vi "build.flowToVarient.vi"(11 "Flow Element":T1) -> (0 "error out":errorcluster, 3 "instructions out":variant[](array[variant])=[variant("stepDoutString"=variant(string ""), "stepFunction"=variant(enum16{"__NO-OP", "_DELAY_LOAD", "_DELAY_COMPARE", "_COMPARE", "_JUMP", "_FINISH", "CLK_COMPARE", "PROC_START", "PROC_STOP", "PROC_ISRUN_IF_OFF", "PROC_ISRUN_LOAD", "_IO_READ_IN", "_IO_WRITE_DOUT", "_IO_COMPARE", "Q_OPEN", "Q_WRITE", "Q_READ"} enum."_IO_WRITE_DOUT"), "stepIoPointer"=variant(string ""), "stepLabel"=variant(string ""), "stepPath"=variant(string ""))])   [LabVIEW 2024]
uses:
  controls/UiStepBuilder.ctl
  controls/type.step-builder.ctl
  controls/typeStepVarients.ctl
  controls/type.StepFunction.ctl
  Polymorphics/variantCtrlStepFunction.vi
  Polymorphics/variantCtrlSetpoint.vi
  Polymorphics/variantCtrlString.vi
  Polymorphics/variantCtrlNumber.vi
  proc.util.validateParamExist.vi
  <vilib>/Utility/error.llb/Clear Errors.vi
  <vilib>/Utility/error.llb/Trim Whitespace.vi
  <vilib>/Utility/error.llb/Trim Whitespace One-Sided.vi
  util.error.create.vi
  Polymorphics/variantCtrlStepPointer.vi
  Polymorphics/variantCtrlStepUserMessage.vi
  Polymorphics/variantCtrlStepPath.vi
  <vilib>/Utility/miscctls.llb/LVPointTypeDef.ctl
panel:
  out "format string":string
  # "UNIT-CHECK(UNIT_INDEX)"
  # "UNIT-DOSE(UNIT_INDEX,DOSE_PUNP,DOSE_TIME)"
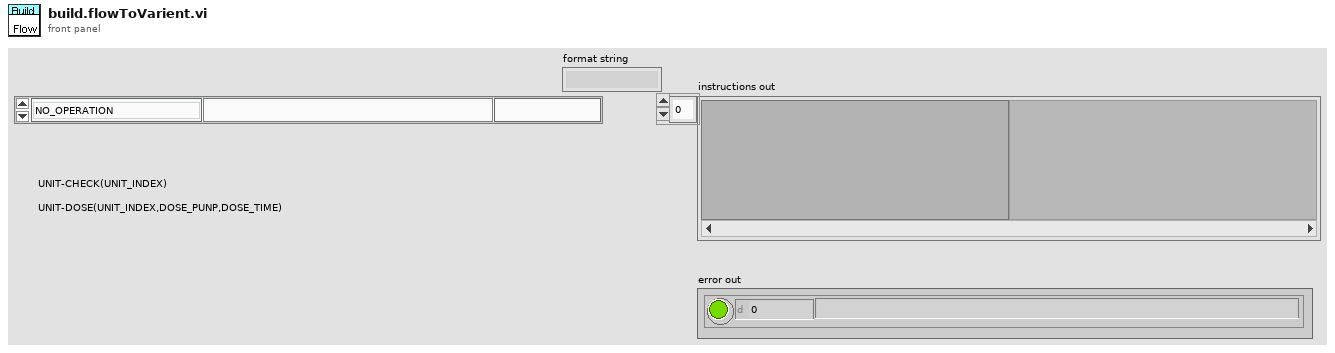
[diagram p1: front panel]
types:
  T1 = typedef "UiStepBuilder.ctl" = cluster{"Step Function":T2, "ParamString":string, "Step Label":string}
  T2 = typedef "type.step-builder.ctl" = enum16{"NO_OPERATION", "DELAY-JUMP", "DELAY", "JUMP", "COMPLETE", "SCHEDULER", "IRR-CHECK", "UNIT-CHECK", "UNIT-SAMPLE", "UNIT-DOSE", "LOG-REPORT", "LOG-MESSAGE", "IO-READ", "IO-READ-MANY", "IO-WRITE", "IO-COMPARE-OUT", "IO-COMPARE-IN", "PROC-START", "PROC-STOP", "PROC-LOAD", "PROC-IS-COMPLETED", "RECORD-MOVE", "GET-RH", "GET-UV", "GET-WD", "GET-WS", "OCS-CHECK", "OCS-RECORD"}
  T3 = typedef "typeStepVarients.ctl" = enum16{"stepNameID", "stepFunction", "stepReport", "stepSetpoint", "stepPointer", "stepProcPointer", "stepIoPointer", "stepIoValue", "stepFilePointer", "stepMessage", "stepTimeString", "stepNumReg", "stepStrReg", "stepSeconds", "stepUnitDoseParams", "stepUnitIndex"}
  T4 = typedef "LVPointTypeDef.ctl" = cluster{"Horizontal":i16, "Vertical":i16}
  T5 = typedef "type.StepFunction.ctl" = enum16{"__NO-OP", "_DELAY_LOAD", "_DELAY_COMPARE", "_JUMP", "_COMPLETE", "_COMPARE", "_LOG_MESSAGE", "_LOG_LAST_REPORT", "_SCHEDULE", "_SCHED_DAILY", "CLK_COMPARE", "PROC_START", "PROC_STOP", "PROC_LOAD", "PROC_COMPLETION_CHECK", "PROC_COMPLETION_LOAD", "_IO_READ", "_IO_READ_MANY", "_IO_WRITE", "_IO_WRITE_BY_REG", "_IO_GET_OUTPUT", "_OCS_CHECK", "_OCS_RECORD", "_GET_RH", "_GET_ACC_UV", "_GET_WD", "_GET_WS", "_REC_DELETE", "_REC_MOVE", "_REC_COPY", "_IRR_CHECK", "UNIT_CHECK", "UNIT_SAMPLE", "UNIT_DOSE"}
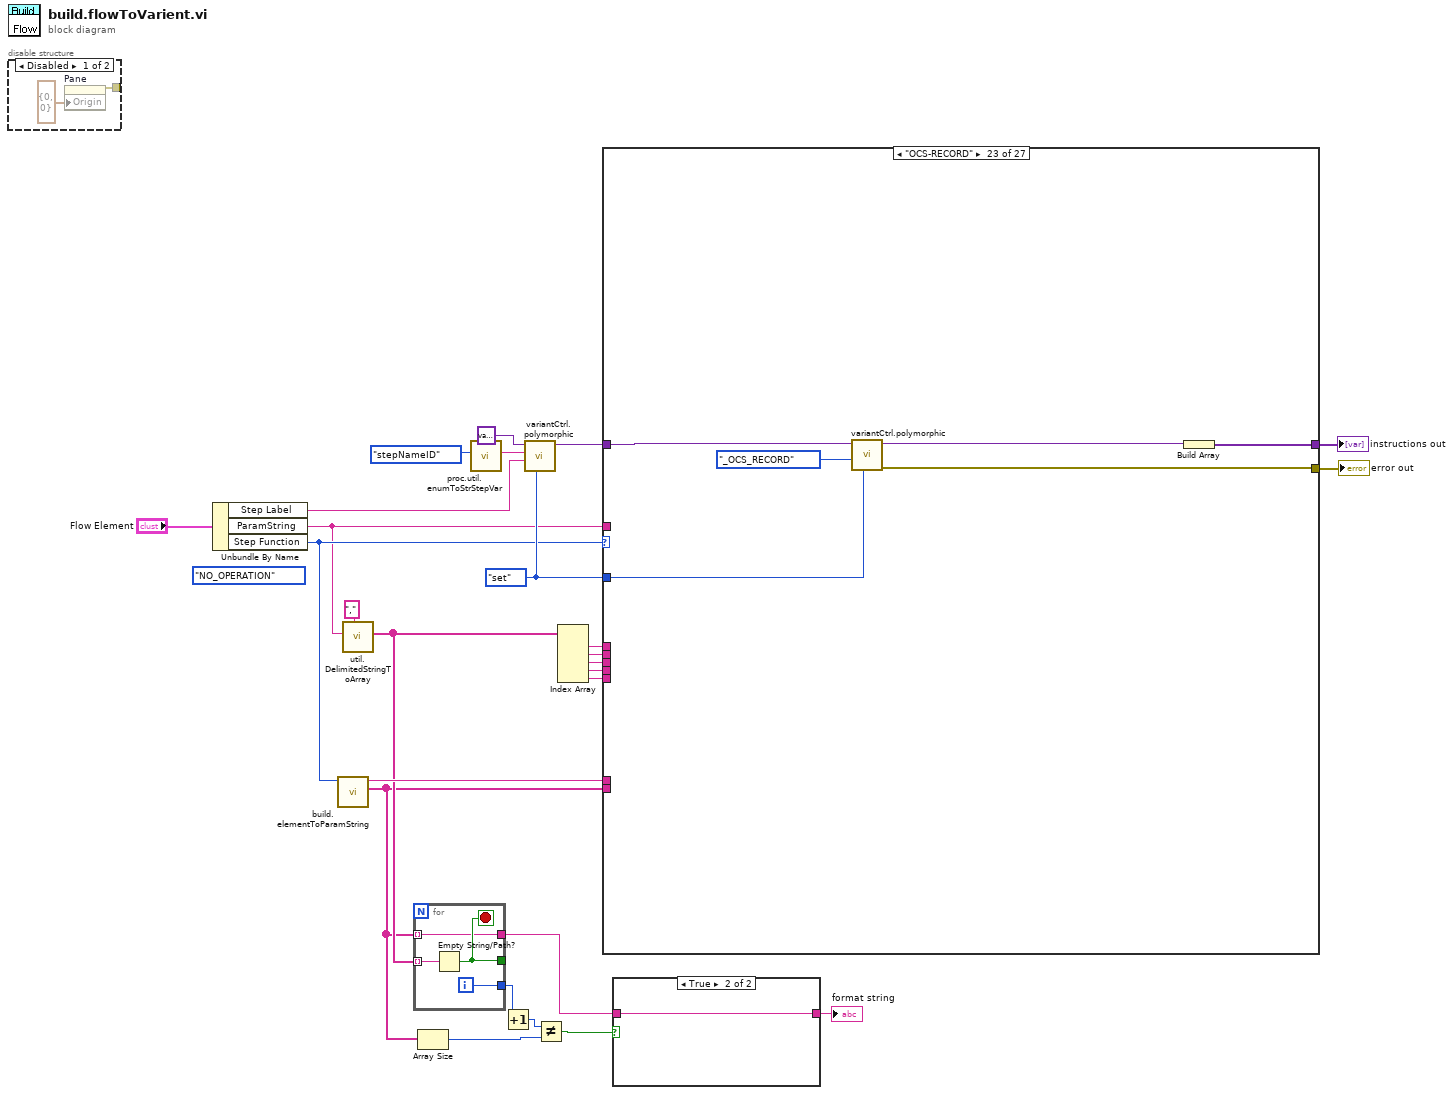
[diagram p0: block diagram]
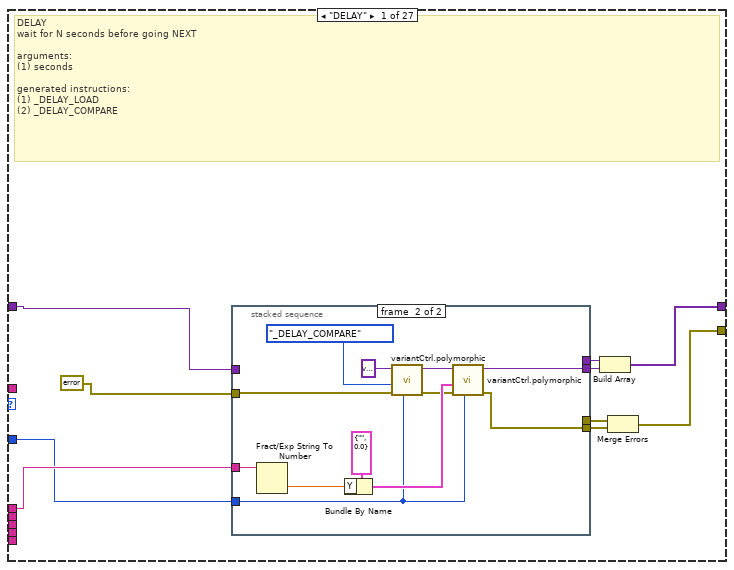
[diagram p3: hidden frame]
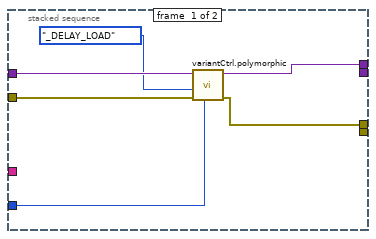
[diagram p4: hidden frame]
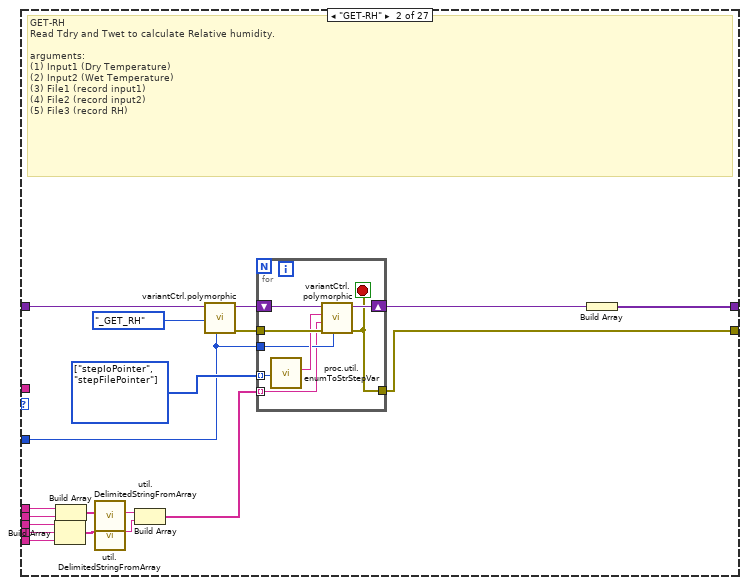
[diagram p5: hidden frame]
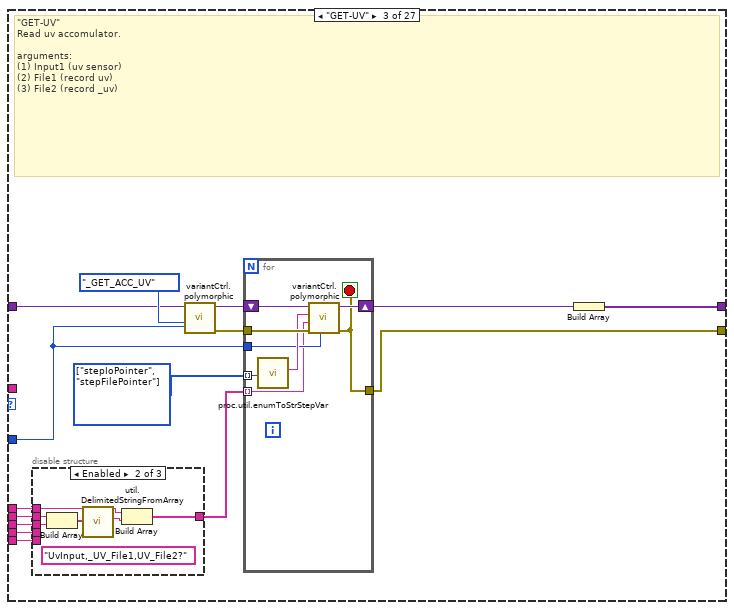
[diagram p6: hidden frame]
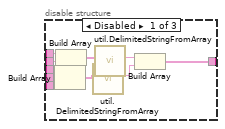
[diagram p7: hidden frame]
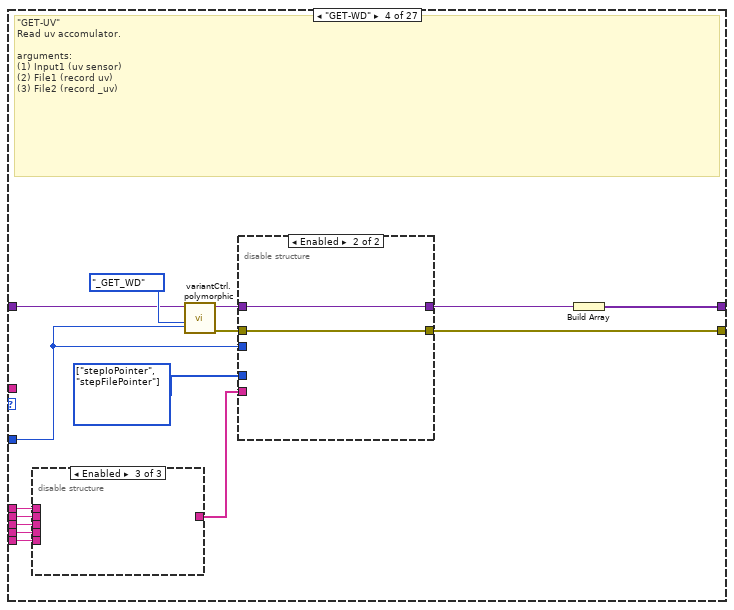
[diagram p9: hidden frame]
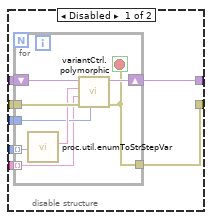
[diagram p10: hidden frame]
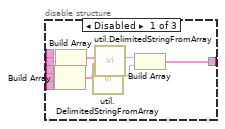
[diagram p11: hidden frame]
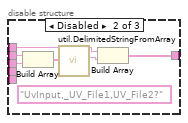
[diagram p12: hidden frame]
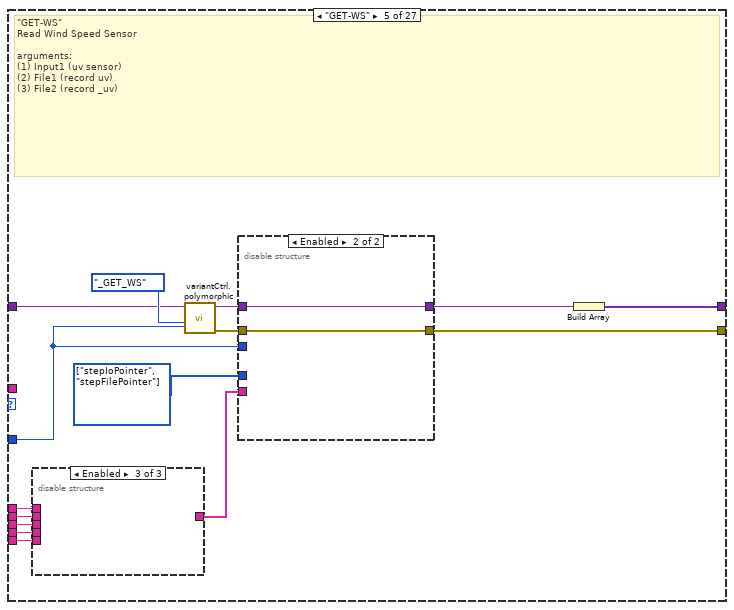
[diagram p13: hidden frame]
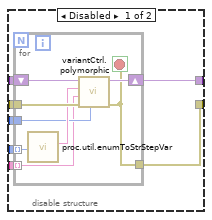
[diagram p14: hidden frame]
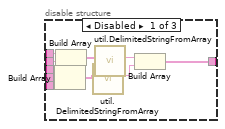
[diagram p15: hidden frame]
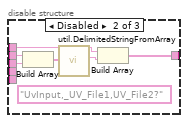
[diagram p16: hidden frame]
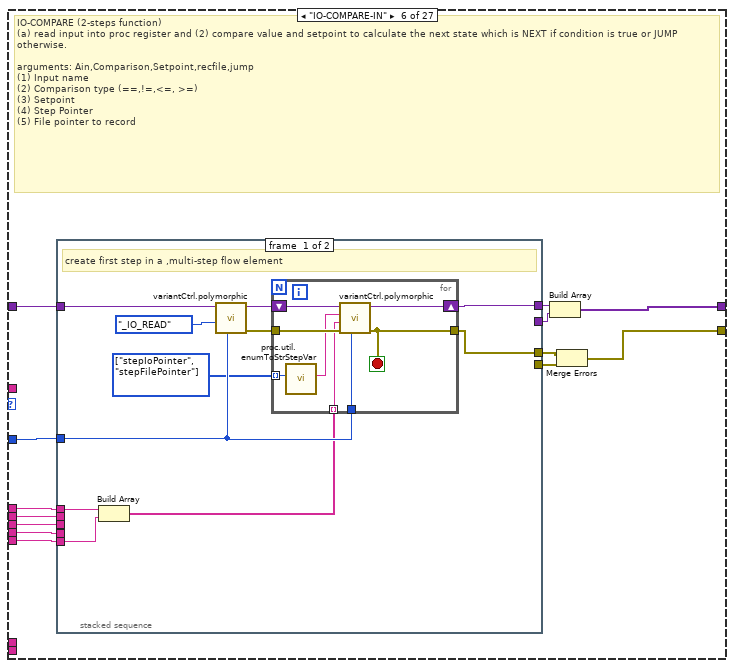
[diagram p17: hidden frame]
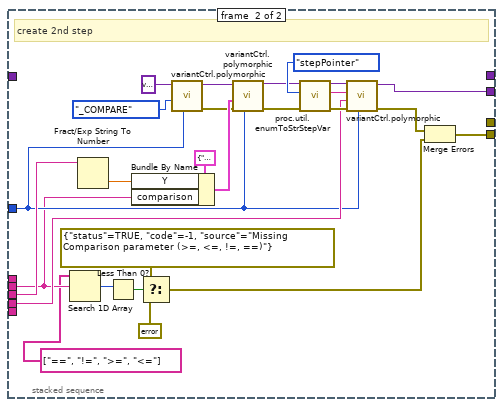
[diagram p18: hidden frame]
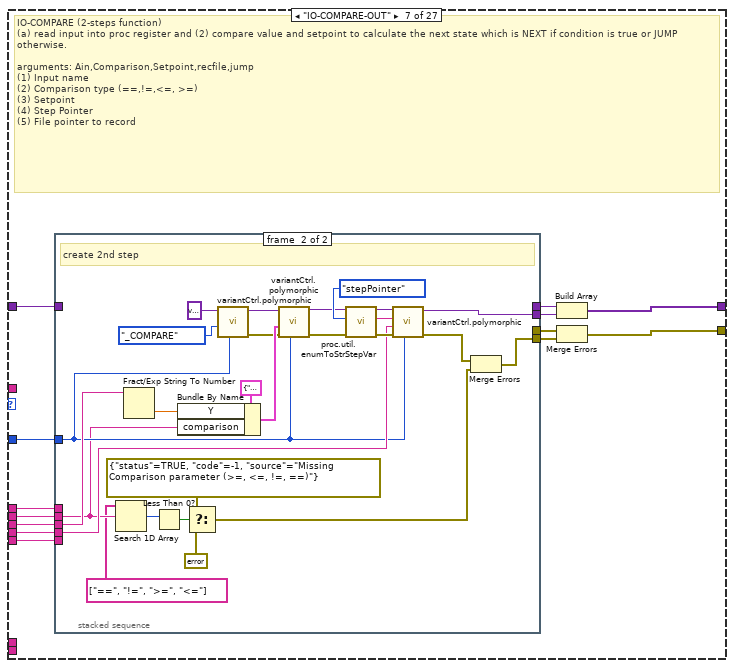
[diagram p19: hidden frame]
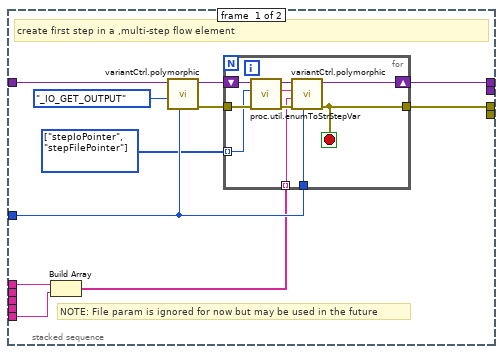
[diagram p20: hidden frame]
diagram:
  (unwired) type.step-builder."NO_OPERATION" ("Step Function")
  w16 = enum16{"get", "set"}."set" ("get/set")
  n1 = disable-structure shown="Disabled" {
    disable-tunnel: [w27 _] -> _
    frame Disabled {
      n2 = property on="Pane" class="Pane"("Origin"=T4 {"Horizontal"=0, "Vertical"=0}) -> (error out=w27:errorcluster)  [unwired: 2 in, 1 out]
    }
    frame Enabled {
    }
  }
  n3 = Unbundle By Name("Flow Element") -> ("Step Label"=w23:string, "ParamString"=w1:string, "Step Function"=w12:T2)
  n4 = call "build.elementToParamString.vi"("UiStepFunction"=w12) -> ("params"=w6:string[], "source"=w11:string)  [unwired: 9 in]
  n5 = call "util.DelimitedStringToArray.vi"("delimiter (,)"=",", "delimitaed string"=w1) -> ("array out"=w10:string[])  [unwired: 9 in]
  n6 = for {
    tunnel: w10 -> [w32] mode=indexing
    tunnel: [w31] -> w9
    tunnel: [w30] -> _
    tunnel: w6 -> [w29] mode=indexing
    tunnel: [w29] -> w4
    i -> [w31]
    stop <- w30 stop-if-true
    n7 = Empty String/Path?(string/path=w32) -> (empty?=w30:bool)
  }
  n8 = Array Size(array=w6) -> (size(s)=w8:i32)
  n9 = call "proc.util.enumToStrStepVar.vi"("Step var"=typeStepVarients."stepNameID") -> ("String"=w20:string)  [unwired: 10 in]
  n10 = Increment(x=w9) -> (x+1=w7:i32)
  n11 = call-poly "variantCtrl.polymorphic.vi"("menu in (get)"=w16, "String Value"=w23, "name in"=w20, "Step in"=variant ("stepElement _DELAY_LOAD")) -> ("Step out"=w19:variant)  [unwired: 4 in, 3 out]
  n12 = Not Equal?(x=w7, y=w8) -> (x != y?=w5:bool)
  n13 = Index Array(array=w10) -> (element #1=w18:string, element #2=w17:string, element #3=w15:string, element #4=w14:string, element #5=w13:string)  [unwired: 5 in]
  n14 = case shown="\"OCS-RECORD\"" w12 {
    selector: w12 -> [_ _ _ _ _ _ _ _ _ _ _ _ _ _ _ _ _ _ _ _ _ _ _ _ _ _ w655]
    tunnel: [w39 w79 w102 w141 w189 w235 w291 w341 w366 w398 w415 w421 w433 w450 w459 w490 w501 w512 w528 w555 w569 w585 w591 w603 w617 w647 variant[] []] -> w26
    tunnel: [w42 w75 w97 w136 w184 w234 w290 w340 w365 w397 w408 w416 w424 w446 w454 w483 w495 w505 w523 w554 w568 w582 w588 w602 w616 w649 w652] -> w25
    tunnel: w19 -> [w41 w72 w94 w133 w181 w233 w289 w337 w362 w395 w411 w419 w432 w449 w453 w480 w491 w502 w520 w553 w567 w584 w590 w601 w615 w648 _]
    tunnel: w16 -> [w33 w74 w96 w135 w183 w232 w288 w339 w364 _ w410 w418 w423 w448 w452 w482 w494 w504 w522 w552 w566 w583 w589 w600 w614 w628 _]
    tunnel: w18 -> [w40 w73 w95 w134 w182 w231 w287 w338 w363 w396 w407 _ w428 w442 w451 w481 w492 w503 w521 w545 w557 _ _ _ w605 w629 _]
    tunnel: w17 -> [_ w70 w92 w131 w179 w230 w286 w335 _ w392 _ _ w422 _ _ _ _ _ w518 _ _ _ _ _ _ w646 _]
    tunnel: w15 -> [_ w67 w91 w130 w178 w229 w285 _ _ w391 _ _ _ _ _ _ _ _ w517 _ _ _ _ _ _ w645 _]
    tunnel: w14 -> [_ w66 w90 w129 w177 w228 w284 _ _ _ _ _ _ _ _ _ _ _ w516 _ _ _ _ _ _ _ _]
    tunnel: w13 -> [_ w65 w89 w128 w176 w227 w283 _ _ _ _ _ _ _ _ _ _ _ w515 _ _ _ _ _ _ _ _]
    tunnel: w11 -> [_ _ _ _ _ _ _ _ _ _ _ _ _ _ _ _ _ _ _ _ _ _ _ _ _ _ _]
    tunnel: w6 -> [_ _ _ _ _ _ _ _ _ _ _ _ _ _ _ _ _ _ _ _ _ _ _ _ _ _ _]
    tunnel: w1 -> [_ _ _ _ _ _ _ _ _ _ _ _ _ _ _ _ _ _ _ _ _ _ _ w592 _ _ _]
    frame "DELAY" {
      # "DELAY\nwait for N seconds before going NEXT\n\narguments:\n(1) seconds\n\ngenerated instructions:\n(1) _DELAY_LOAD\n(2) _DELAY_COMPARE"
      n15 = stacked-sequence {
        tunnel: [w46 _] -> w37
        tunnel: [_ w51] -> w36
        tunnel: [_ w59] -> w35
        tunnel: [w45 _] -> w34
        tunnel: w40 -> [_ w58]
        tunnel: w41 -> [w48 _]
        tunnel: w33 -> [w47 w54]
        tunnel: errorcluster {"status"=FALSE, "code"=0, "source"=""} ("error in") -> [w43 w49]
        frame #0 {
          n16 = call-poly "variantCtrl.polymorphic.vi"("menu in (get)"=w47, "error in"=w43, "StepFunction"=type.StepFunction."_DELAY_LOAD" ("Operation out"), "variant in"=w48) -> ("error out"=w45:errorcluster, "variant out"=w46:variant)  [unwired: 4 in, 2 out]
        }
        frame #1 {
          n17 = Fract/Exp String To Number(string=w58) -> (number=w57:dbl)  [unwired: 3 in, 1 out]
          n18 = Bundle By Name(cluster=cluster{"comparison":string, "Y":dbl} {"comparison"="", "Y"=0.0} ("setpoint 2"), "Y"=w57) -> (w60:cluster{"comparison":string, "Y":dbl})
          n19 = call-poly "variantCtrl.polymorphic.vi"("menu in (get)"=w54, "error in"=w49, "StepFunction"=type.StepFunction."_DELAY_COMPARE" ("Operation out"), "variant in"=variant ("stepElement _DELAY_LOAD")) -> ("error out"=w55:errorcluster, "variant out"=w56:variant)  [unwired: 4 in, 2 out]
          n20 = call-poly "variantCtrl.polymorphic.vi"("get/set"=w54, "error in"=w55, "setpoint"=w60, "procElement in in"=w56) -> ("error out"=w59:errorcluster, "procElement out"=w51:variant)  [unwired: 4 in, 2 out]
        }
      }
      n21 = Build Array(w37, w36) -> (w39:variant[])
      n22 = Merge Errors(w34, w35) -> (w42:errorcluster)
    }
    frame "GET-RH" {
      w76 = T3[] [enum."stepIoPointer", enum."stepFilePointer"] items=["stepNameID", "stepFunction", "stepReport", "stepSetpoint", "stepPointer", "stepProcPointer", "stepIoPointer", "stepIoValue", "stepFilePointer", "stepMessage", "stepTimeString", "stepNumReg", "stepStrReg", "stepSeconds", "stepUnitDoseParams", "stepUnitIndex"] ("Step var")
      # "GET-RH\nRead Tdry and Twet to calculate Relative humidity.\n\narguments:\n(1) Input1 (Dry Temperature)\n(2) Input2 (Wet Temperature)\n(3) File1 (record input1)\n(4) File2 (record input2)\n(5) File3 (record RH)"
      n23 = Build Array(w67, w66, w65) -> (w64:string[])
      n24 = Build Array(w73, w70) -> (w69:string[])
      n25 = call "util.DelimitedStringFromArray.vi"("params array in"=w69) -> ("delimited string out"=w68:string)  [unwired: 10 in]
      n26 = call "util.DelimitedStringFromArray.vi"("params array in"=w64) -> ("delimited string out"=w62:string)  [unwired: 10 in]
      n27 = Build Array(w68, w62) -> (w63:string[])
      n28 = call-poly "variantCtrl.polymorphic.vi"("menu in (get)"=w74, "StepFunction"=type.StepFunction."_GET_RH" ("Operation out"), "variant in"=w72) -> ("error out"=w78:errorcluster, "variant out"=w77:variant)  [unwired: 5 in, 2 out]
      n29 = for {
        tunnel: w76 -> [w85] mode=indexing
        tunnel: w74 -> [w83]
        tunnel: w63 -> [w82] mode=indexing
        shift-right: [w81] -> w71
        shift-left: w77 -> [w86]
        tunnel: w78 -> [w87]
        tunnel: [w80] -> w75
        stop <- w80 stop-if-true
        n30 = call "proc.util.enumToStrStepVar.vi"("Step var"=w85) -> ("String"=w84:string)  [unwired: 10 in]
        n31 = call-poly "variantCtrl.polymorphic.vi"("menu in (get)"=w83, "error in"=w87, "String Value"=w82, "name in"=w84, "Step in"=w86) -> ("error out"=w80:errorcluster, "Step out"=w81:variant)  [unwired: 3 in, 2 out]
      }
      n32 = Build Array(w71) -> (w79:variant[])
    }
    frame "GET-UV" {
      w98 = T3[] [enum."stepIoPointer", enum."stepFilePointer"] items=["stepNameID", "stepFunction", "stepReport", "stepSetpoint", "stepPointer", "stepProcPointer", "stepIoPointer", "stepIoValue", "stepFilePointer", "stepMessage", "stepTimeString", "stepNumReg", "stepStrReg", "stepSeconds", "stepUnitDoseParams", "stepUnitIndex"] ("Step var")
      # "\"GET-UV\" \nRead uv accomulator.\n\narguments:\n(1) Input1 (uv sensor)\n(2) File1 (record uv)\n(3) File2 (record _uv)"
      n33 = disable-structure shown="Enabled" {
        disable-tunnel: w95 -> [w112 w114 _]
        disable-tunnel: w92 -> [w111 w113 _]
        disable-tunnel: w91 -> [w108 w118 _]
        disable-tunnel: w90 -> [w107 _ _]
        disable-tunnel: w89 -> [w106 _ _]
        disable-tunnel: [w104 w116 _] -> w88
        frame Disabled {
          n34 = Build Array(w108, w107, w106) -> (w105:string[])
          n35 = Build Array(w112, w111) -> (w110:string[])
          n36 = call "util.DelimitedStringFromArray.vi"("params array in"=w105) -> ("delimited string out"=w103:string)  [unwired: 10 in]
          n37 = call "util.DelimitedStringFromArray.vi"("params array in"=w110) -> ("delimited string out"=w109:string)  [unwired: 10 in]
          n38 = Build Array(w109, w103) -> (w104:string[])
        }
        frame Enabled {
          (unwired) "UvInput,_UV_File1,UV_File2?" ("source")
          n39 = Build Array(w113, w118) -> (w117:string[])
          n40 = call "util.DelimitedStringFromArray.vi"("params array in"=w117) -> ("delimited string out"=w115:string)  [unwired: 10 in]
          n41 = Build Array(w114, w115) -> (w116:string[])
        }
        frame Disabled {
        }
      }
      n42 = call-poly "variantCtrl.polymorphic.vi"("menu in (get)"=w96, "StepFunction"=type.StepFunction."_GET_ACC_UV" ("Operation out"), "variant in"=w94) -> ("error out"=w101:errorcluster, "variant out"=w100:variant)  [unwired: 5 in, 2 out]
      n43 = for {
        tunnel: w98 -> [w124] mode=indexing
        tunnel: w96 -> [w122]
        tunnel: w88 -> [w121] mode=indexing
        shift-right: [w120] -> w93
        shift-left: w100 -> [w125]
        tunnel: w101 -> [w126]
        tunnel: [w119] -> w97
        stop <- w119 stop-if-true
        n44 = call "proc.util.enumToStrStepVar.vi"("Step var"=w124) -> ("String"=w123:string)  [unwired: 10 in]
        n45 = call-poly "variantCtrl.polymorphic.vi"("menu in (get)"=w122, "error in"=w126, "String Value"=w121, "name in"=w123, "Step in"=w125) -> ("error out"=w119:errorcluster, "Step out"=w120:variant)  [unwired: 3 in, 2 out]
      }
      n46 = Build Array(w93) -> (w102:variant[])
    }
    frame "GET-WD" {
      w137 = T3[] [enum."stepIoPointer", enum."stepFilePointer"] items=["stepNameID", "stepFunction", "stepReport", "stepSetpoint", "stepPointer", "stepProcPointer", "stepIoPointer", "stepIoValue", "stepFilePointer", "stepMessage", "stepTimeString", "stepNumReg", "stepStrReg", "stepSeconds", "stepUnitDoseParams", "stepUnitIndex"] ("Step var")
      # "\"GET-UV\" \nRead uv accomulator.\n\narguments:\n(1) Input1 (uv sensor)\n(2) File1 (record uv)\n(3) File2 (record _uv)"
      n47 = disable-structure shown="Enabled" {
        disable-tunnel: w134 -> [w168 w170 _]
        disable-tunnel: w131 -> [w167 w169 _]
        disable-tunnel: w130 -> [w164 w174 _]
        disable-tunnel: w129 -> [w163 _ _]
        disable-tunnel: w128 -> [w162 _ _]
        disable-tunnel: [w160 w172 _] -> w127
        frame Disabled {
          n48 = Build Array(w164, w163, w162) -> (w161:string[])
          n49 = Build Array(w168, w167) -> (w166:string[])
          n50 = call "util.DelimitedStringFromArray.vi"("params array in"=w161) -> ("delimited string out"=w159:string)  [unwired: 10 in]
          n51 = call "util.DelimitedStringFromArray.vi"("params array in"=w166) -> ("delimited string out"=w165:string)  [unwired: 10 in]
          n52 = Build Array(w165, w159) -> (w160:string[])
        }
        frame Disabled {
          (unwired) "UvInput,_UV_File1,UV_File2?" ("source")
          n53 = Build Array(w169, w174) -> (w173:string[])
          n54 = call "util.DelimitedStringFromArray.vi"("params array in"=w173) -> ("delimited string out"=w171:string)  [unwired: 10 in]
          n55 = Build Array(w170, w171) -> (w172:string[])
        }
        frame Enabled {
        }
      }
      n56 = call-poly "variantCtrl.polymorphic.vi"("menu in (get)"=w135, "StepFunction"=type.StepFunction."_GET_WD" ("Operation out"), "variant in"=w133) -> ("error out"=w140:errorcluster, "variant out"=w139:variant)  [unwired: 5 in, 2 out]
      n57 = disable-structure shown="Enabled" {
        disable-tunnel: w140 -> [w148 w157]
        disable-tunnel: w139 -> [w147 w158]
        disable-tunnel: w137 -> [w146 _]
        disable-tunnel: [w145 w157] -> w136
        disable-tunnel: w135 -> [w144 _]
        disable-tunnel: [w143 w158] -> w132
        disable-tunnel: w127 -> [w142 _]
        frame Disabled {
          n58 = for {
            tunnel: w146 -> [w154] mode=indexing
            tunnel: w144 -> [w152]
            tunnel: w142 -> [w151] mode=indexing
            shift-right: [w150] -> w143
            shift-left: w147 -> [w155]
            tunnel: w148 -> [w156]
            tunnel: [w149] -> w145
            stop <- w149 stop-if-true
            n59 = call "proc.util.enumToStrStepVar.vi"("Step var"=w154) -> ("String"=w153:string)  [unwired: 10 in]
            n60 = call-poly "variantCtrl.polymorphic.vi"("menu in (get)"=w152, "error in"=w156, "String Value"=w151, "name in"=w153, "Step in"=w155) -> ("error out"=w149:errorcluster, "Step out"=w150:variant)  [unwired: 3 in, 2 out]
          }
        }
        frame Enabled {
        }
      }
      n61 = Build Array(w132) -> (w141:variant[])
    }
    frame "GET-WS" {
      w185 = T3[] [enum."stepIoPointer", enum."stepFilePointer"] items=["stepNameID", "stepFunction", "stepReport", "stepSetpoint", "stepPointer", "stepProcPointer", "stepIoPointer", "stepIoValue", "stepFilePointer", "stepMessage", "stepTimeString", "stepNumReg", "stepStrReg", "stepSeconds", "stepUnitDoseParams", "stepUnitIndex"] ("Step var")
      # "\"GET-WS\"  \nRead Wind Speed Sensor \n\narguments:\n(1) Input1 (uv sensor)\n(2) File1 (record uv)\n(3) File2 (record _uv)"
      n62 = disable-structure shown="Enabled" {
        disable-tunnel: w182 -> [w216 w218 _]
        disable-tunnel: w179 -> [w215 w217 _]
        disable-tunnel: w178 -> [w212 w222 _]
        disable-tunnel: w177 -> [w211 _ _]
        disable-tunnel: w176 -> [w210 _ _]
        disable-tunnel: [w208 w220 _] -> w175
        frame Disabled {
          n63 = Build Array(w212, w211, w210) -> (w209:string[])
          n64 = Build Array(w216, w215) -> (w214:string[])
          n65 = call "util.DelimitedStringFromArray.vi"("params array in"=w209) -> ("delimited string out"=w207:string)  [unwired: 10 in]
          n66 = call "util.DelimitedStringFromArray.vi"("params array in"=w214) -> ("delimited string out"=w213:string)  [unwired: 10 in]
          n67 = Build Array(w213, w207) -> (w208:string[])
        }
        frame Disabled {
          (unwired) "UvInput,_UV_File1,UV_File2?" ("source")
          n68 = Build Array(w217, w222) -> (w221:string[])
          n69 = call "util.DelimitedStringFromArray.vi"("params array in"=w221) -> ("delimited string out"=w219:string)  [unwired: 10 in]
          n70 = Build Array(w218, w219) -> (w220:string[])
        }
        frame Enabled {
        }
      }
      n71 = call-poly "variantCtrl.polymorphic.vi"("menu in (get)"=w183, "StepFunction"=type.StepFunction."_GET_WS" ("Operation out"), "variant in"=w181) -> ("error out"=w188:errorcluster, "variant out"=w187:variant)  [unwired: 5 in, 2 out]
      n72 = disable-structure shown="Enabled" {
        disable-tunnel: w188 -> [w196 w205]
        disable-tunnel: w187 -> [w195 w206]
        disable-tunnel: w185 -> [w194 _]
        disable-tunnel: [w193 w205] -> w184
        disable-tunnel: w183 -> [w192 _]
        disable-tunnel: [w191 w206] -> w180
        disable-tunnel: w175 -> [w190 _]
        frame Disabled {
          n73 = for {
            tunnel: w194 -> [w202] mode=indexing
            tunnel: w192 -> [w200]
            tunnel: w190 -> [w199] mode=indexing
            shift-right: [w198] -> w191
            shift-left: w195 -> [w203]
            tunnel: w196 -> [w204]
            tunnel: [w197] -> w193
            stop <- w197 stop-if-true
            n74 = call "proc.util.enumToStrStepVar.vi"("Step var"=w202) -> ("String"=w201:string)  [unwired: 10 in]
            n75 = call-poly "variantCtrl.polymorphic.vi"("menu in (get)"=w200, "error in"=w204, "String Value"=w199, "name in"=w201, "Step in"=w203) -> ("error out"=w197:errorcluster, "Step out"=w198:variant)  [unwired: 3 in, 2 out]
          }
        }
        frame Enabled {
        }
      }
      n76 = Build Array(w180) -> (w189:variant[])
    }
    frame "IO-COMPARE-IN" {
      # "IO-COMPARE (2-steps function)\n(a) read input into proc register and (2) compare value and setpoint to calculate the next state which is NEXT if condition is true or JUMP otherwise. \n\narguments: Ain,Comparison,Setpoint,recfile,jump\n(1) Input name\n(2) Comparison type (==,!=,<=, >=)\n(3) Setpoint\n(4) Step Pointer\n(5) File pointer to record"
      n77 = stacked-sequence {
        tunnel: [w243 _] -> w226
        tunnel: w231 -> [w244 _]
        tunnel: w233 -> [w246 _]
        tunnel: w232 -> [w245 w262]
        tunnel: w230 -> [_ w261]
        tunnel: w229 -> [_ w271]
        tunnel: w228 -> [_ w263]
        tunnel: w227 -> [w236 _]
        tunnel: [_ w257] -> w225
        tunnel: [w237 _] -> w224
        tunnel: [_ w256] -> w223
        frame #0 {
          w239 = T3[] [enum."stepIoPointer", enum."stepFilePointer"] items=["stepNameID", "stepFunction", "stepReport", "stepSetpoint", "stepPointer", "stepProcPointer", "stepIoPointer", "stepIoValue", "stepFilePointer", "stepMessage", "stepTimeString", "stepNumReg", "stepStrReg", "stepSeconds", "stepUnitDoseParams", "stepUnitIndex"] ("Step var")
          # "create first step in a ,multi-step flow element"
          n78 = Build Array(w244, w236) -> (w238:string[])
          n79 = call-poly "variantCtrl.polymorphic.vi"("menu in (get)"=w245, "StepFunction"=type.StepFunction."_IO_READ" ("Operation out"), "variant in"=w246) -> ("error out"=w242:errorcluster, "variant out"=w241:variant)  [unwired: 5 in, 2 out]
          n80 = for {
            tunnel: w239 -> [w252] mode=indexing
            tunnel: w245 -> [w250]
            tunnel: w238 -> [w249] mode=indexing
            shift-right: [w248] -> w237
            shift-left: w241 -> [w253]
            tunnel: w242 -> [w254]
            tunnel: [w247] -> w243
            stop <- w247 stop-if-true
            n81 = call "proc.util.enumToStrStepVar.vi"("Step var"=w252) -> ("String"=w251:string)  [unwired: 10 in]
            n82 = call-poly "variantCtrl.polymorphic.vi"("menu in (get)"=w250, "error in"=w254, "String Value"=w249, "name in"=w251, "Step in"=w253) -> ("error out"=w247:errorcluster, "Step out"=w248:variant)  [unwired: 3 in, 2 out]
          }
        }
        frame #1 {
          # "create 2nd step"
          n83 = Search 1D Array(1D array=string[] ["==", "!=", ">=", "<="] ("source"), element=w261) -> (index of element=w260:i32)  [unwired: 1 in]
          n84 = Fract/Exp String To Number(string=w271) -> (number=w276:dbl)  [unwired: 3 in, 1 out]
          n85 = Less Than 0?(x=w260) -> (x < 0?=w259:bool)
          n86 = Bundle By Name(cluster=cluster{"comparison":string, "Y":dbl} {"comparison"="", "Y"=0.0} ("setpoint"), "Y"=w276, "comparison"=w261) -> (w278:cluster{"comparison":string, "Y":dbl})
          n87 = Select(t=errorcluster {"status"=TRUE, "code"=-1, "source"="Missing Comparison parameter (>=, <=, !=, ==)"} ("error out"), s=w259, f=errorcluster {"status"=FALSE, "code"=0, "source"=""}) -> (s? t:f=w269:errorcluster)
          n88 = call-poly "variantCtrl.polymorphic.vi"("menu in (get)"=w262, "StepFunction"=type.StepFunction."_COMPARE" ("Operation out"), "variant in"=variant ("stepElement _DELAY_LOAD")) -> ("error out"=w274:errorcluster, "variant out"=w275:variant)  [unwired: 5 in, 2 out]
          n89 = call-poly "variantCtrl.polymorphic.vi"("get/set"=w262, "error in"=w274, "setpoint"=w278, "procElement in in"=w275) -> ("error out"=w264:errorcluster, "procElement out"=w266:variant)  [unwired: 4 in, 2 out]
          n90 = call "proc.util.enumToStrStepVar.vi"("Step var"=typeStepVarients."stepPointer") -> ("String"=w267:string)  [unwired: 10 in]
          n91 = call-poly "variantCtrl.polymorphic.vi"("menu in (get)"=w262, "error in"=w264, "String Value"=w263, "name in"=w267, "Step in"=w266) -> ("error out"=w265:errorcluster, "Step out"=w257:variant)  [unwired: 3 in, 2 out]
          n92 = Merge Errors(w265, w269) -> (w256:errorcluster)
        }
      }
      n93 = Build Array(w224, w225) -> (w235:variant[])
      n94 = Merge Errors(w226, w223) -> (w234:errorcluster)
    }
    frame "IO-COMPARE-OUT" {
      # "IO-COMPARE (2-steps function)\n(a) read input into proc register and (2) compare value and setpoint to calculate the next state which is NEXT if condition is true or JUMP otherwise. \n\narguments: Ain,Comparison,Setpoint,recfile,jump\n(1) Input name\n(2) Comparison type (==,!=,<=, >=)\n(3) Setpoint\n(4) Step Pointer\n(5) File pointer to record"
      n95 = stacked-sequence {
        tunnel: [w299 _] -> w282
        tunnel: w287 -> [w300 _]
        tunnel: w289 -> [w302 _]
        tunnel: w288 -> [w301 w318]
        tunnel: w286 -> [_ w317]
        tunnel: w285 -> [_ w327]
        tunnel: w284 -> [_ w319]
        tunnel: w283 -> [w292 _]
        tunnel: [_ w313] -> w281
        tunnel: [w293 _] -> w280
        tunnel: [_ w312] -> w279
        frame #0 {
          w295 = T3[] [enum."stepIoPointer", enum."stepFilePointer"] items=["stepNameID", "stepFunction", "stepReport", "stepSetpoint", "stepPointer", "stepProcPointer", "stepIoPointer", "stepIoValue", "stepFilePointer", "stepMessage", "stepTimeString", "stepNumReg", "stepStrReg", "stepSeconds", "stepUnitDoseParams", "stepUnitIndex"] ("Step var")
          # "NOTE: File param is ignored for now but may be used in the future"
          # "create first step in a ,multi-step flow element"
          n96 = Build Array(w300, w292) -> (w294:string[])
          n97 = call-poly "variantCtrl.polymorphic.vi"("menu in (get)"=w301, "StepFunction"=type.StepFunction."_IO_GET_OUTPUT" ("Operation out"), "variant in"=w302) -> ("error out"=w298:errorcluster, "variant out"=w297:variant)  [unwired: 5 in, 2 out]
          n98 = for {
            tunnel: w295 -> [w308] mode=indexing
            tunnel: w301 -> [w306]
            tunnel: w294 -> [w305] mode=indexing
            shift-right: [w304] -> w293
            shift-left: w297 -> [w309]
            tunnel: w298 -> [w310]
            tunnel: [w303] -> w299
            stop <- w303 stop-if-true
            n99 = call "proc.util.enumToStrStepVar.vi"("Step var"=w308) -> ("String"=w307:string)  [unwired: 10 in]
            n100 = call-poly "variantCtrl.polymorphic.vi"("menu in (get)"=w306, "error in"=w310, "String Value"=w305, "name in"=w307, "Step in"=w309) -> ("error out"=w303:errorcluster, "Step out"=w304:variant)  [unwired: 3 in, 2 out]
          }
        }
        frame #1 {
          # "create 2nd step"
          n101 = Search 1D Array(1D array=string[] ["==", "!=", ">=", "<="] ("source"), element=w317) -> (index of element=w316:i32)  [unwired: 1 in]
          n102 = Fract/Exp String To Number(string=w327) -> (number=w332:dbl)  [unwired: 3 in, 1 out]
          n103 = Less Than 0?(x=w316) -> (x < 0?=w315:bool)
          n104 = Bundle By Name(cluster=cluster{"comparison":string, "Y":dbl} {"comparison"="", "Y"=0.0} ("setpoint"), "Y"=w332, "comparison"=w317) -> (w334:cluster{"comparison":string, "Y":dbl})
          n105 = Select(t=errorcluster {"status"=TRUE, "code"=-1, "source"="Missing Comparison parameter (>=, <=, !=, ==)"} ("error out"), s=w315, f=errorcluster {"status"=FALSE, "code"=0, "source"=""}) -> (s? t:f=w325:errorcluster)
          n106 = call-poly "variantCtrl.polymorphic.vi"("menu in (get)"=w318, "StepFunction"=type.StepFunction."_COMPARE" ("Operation out"), "variant in"=variant ("stepElement _DELAY_LOAD")) -> ("error out"=w330:errorcluster, "variant out"=w331:variant)  [unwired: 5 in, 2 out]
          n107 = call-poly "variantCtrl.polymorphic.vi"("get/set"=w318, "error in"=w330, "setpoint"=w334, "procElement in in"=w331) -> ("error out"=w320:errorcluster, "procElement out"=w322:variant)  [unwired: 4 in, 2 out]
          n108 = call "proc.util.enumToStrStepVar.vi"("Step var"=typeStepVarients."stepPointer") -> ("String"=w323:string)  [unwired: 10 in]
          n109 = call-poly "variantCtrl.polymorphic.vi"("menu in (get)"=w318, "error in"=w320, "String Value"=w319, "name in"=w323, "Step in"=w322) -> ("error out"=w321:errorcluster, "Step out"=w313:variant)  [unwired: 3 in, 2 out]
          n110 = Merge Errors(w321, w325) -> (w312:errorcluster)
        }
      }
      n111 = Build Array(w280, w281) -> (w291:variant[])
      n112 = Merge Errors(w282, w279) -> (w290:errorcluster)
    }
    frame "IO-READ" {
      # "IO-READ\nread input, save result to procedure register and a record file\n\narguments:\n(1) Input name\n(2) File pointer (file.*) to record"
      n113 = disable-structure shown="Enabled" {
        disable-tunnel: [w348 _] -> w340
        disable-tunnel: w339 -> [w347 _]
        disable-tunnel: w338 -> [w346 _]
        disable-tunnel: w337 -> [w345 _]
        disable-tunnel: [w344 _] -> w336
        disable-tunnel: w335 -> [w342 _]
        frame Enabled {
          w349 = T3[] [enum."stepIoPointer", enum."stepFilePointer"] items=["stepNameID", "stepFunction", "stepReport", "stepSetpoint", "stepPointer", "stepProcPointer", "stepIoPointer", "stepIoValue", "stepFilePointer", "stepMessage", "stepTimeString", "stepNumReg", "stepStrReg", "stepSeconds", "stepUnitDoseParams", "stepUnitIndex"] ("Step var")
          n114 = Build Array(w346, w342) -> (w343:string[])
          n115 = call-poly "variantCtrl.polymorphic.vi"("menu in (get)"=w347, "StepFunction"=type.StepFunction."_IO_READ" ("Operation out"), "variant in"=w345) -> ("error out"=w352:errorcluster, "variant out"=w351:variant)  [unwired: 5 in, 2 out]
          n116 = for {
            tunnel: w349 -> [w358] mode=indexing
            tunnel: w347 -> [w356]
            tunnel: w343 -> [w355] mode=indexing
            shift-right: [w354] -> w344
            shift-left: w351 -> [w359]
            tunnel: w352 -> [w360]
            tunnel: [w353] -> w348
            stop <- w353 stop-if-true
            n117 = call "proc.util.enumToStrStepVar.vi"("Step var"=w358) -> ("String"=w357:string)  [unwired: 10 in]
            n118 = call-poly "variantCtrl.polymorphic.vi"("menu in (get)"=w356, "error in"=w360, "String Value"=w355, "name in"=w357, "Step in"=w359) -> ("error out"=w353:errorcluster, "Step out"=w354:variant)  [unwired: 3 in, 2 out]
          }
        }
        frame Disabled {
        }
      }
      n119 = Build Array(w336) -> (w341:variant[])
    }
    frame "IO-READ-MANY" {
      # "IO-READ\nread input, save result to procedure register and a record file\n\narguments:\n(1) Input name\n(2) File pointer (file.*) to record"
      n120 = disable-structure shown="Enabled" {
        disable-tunnel: [w372 _] -> w365
        disable-tunnel: w364 -> [w371 _]
        disable-tunnel: w363 -> [w370 _]
        disable-tunnel: w362 -> [w369 _]
        disable-tunnel: [w368 _] -> w361
        frame Enabled {
          w373 = T3[] [enum."stepIoPointer"] items=["stepNameID", "stepFunction", "stepReport", "stepSetpoint", "stepPointer", "stepProcPointer", "stepIoPointer", "stepIoValue", "stepFilePointer", "stepMessage", "stepTimeString", "stepNumReg", "stepStrReg", "stepSeconds", "stepUnitDoseParams", "stepUnitIndex"] ("Step var")
          n121 = Build Array(w370) -> (w367:string[])
          n122 = call-poly "variantCtrl.polymorphic.vi"("menu in (get)"=w371, "StepFunction"=type.StepFunction."_IO_READ_MANY" ("Operation out"), "variant in"=w369) -> ("error out"=w376:errorcluster, "variant out"=w375:variant)  [unwired: 5 in, 2 out]
          n123 = for {
            tunnel: w373 -> [w382] mode=indexing
            tunnel: w371 -> [w380]
            tunnel: w367 -> [w379] mode=indexing
            shift-right: [w378] -> w368
            shift-left: w375 -> [w383]
            tunnel: w376 -> [w384]
            tunnel: [w377] -> w372
            stop <- w377 stop-if-true
            n124 = call "proc.util.enumToStrStepVar.vi"("Step var"=w382) -> ("String"=w381:string)  [unwired: 10 in]
            n125 = call-poly "variantCtrl.polymorphic.vi"("menu in (get)"=w380, "error in"=w384, "String Value"=w379, "name in"=w381, "Step in"=w383) -> ("error out"=w377:errorcluster, "Step out"=w378:variant)  [unwired: 3 in, 2 out]
          }
        }
        frame Disabled {
        }
      }
      n126 = Build Array(w361) -> (w366:variant[])
    }
    frame "IO-WRITE" {
      w385 = enum16{"get", "set"}."set" ("get/set")
      w386 = T3[] [enum."stepIoPointer", enum."stepIoValue", enum."stepFilePointer"] items=["stepNameID", "stepFunction", "stepReport", "stepSetpoint", "stepPointer", "stepProcPointer", "stepIoPointer", "stepIoValue", "stepFilePointer", "stepMessage", "stepTimeString", "stepNumReg", "stepStrReg", "stepSeconds", "stepUnitDoseParams", "stepUnitIndex"] ("Step var")
      # "IO-WRITE\nwrite output and save to record file\n\narguments:\n(1) Output name\n(2) Output State (String formated). For digital outputs use \"A:B\" format where A is 0 or 1 representing the boolean state of digital output and B is timeout value in seconds, de-activating the output automatically\n(3) File pointer (file.*) to record"
      n127 = Build Array(w396, w392, w391) -> (w393:string[])
      n128 = call-poly "variantCtrl.polymorphic.vi"("menu in (get)"=w385, "error in"=errorcluster {"status"=FALSE, "code"=0, "source"=""}, "StepFunction"=type.StepFunction."_IO_WRITE" ("Operation out"), "variant in"=w395) -> ("error out"=w389:errorcluster, "variant out"=w388:variant)  [unwired: 4 in, 2 out]
      n129 = for {
        tunnel: w386 -> [w404] mode=indexing
        tunnel: w385 -> [w402]
        tunnel: w393 -> [w401] mode=indexing
        shift-right: [w400] -> w394
        shift-left: w388 -> [w405]
        tunnel: w389 -> [w406]
        tunnel: [w399] -> w397
        stop <- w399 stop-if-true
        n130 = call "proc.util.enumToStrStepVar.vi"("Step var"=w404) -> ("String"=w403:string)  [unwired: 10 in]
        n131 = call-poly "variantCtrl.polymorphic.vi"("menu in (get)"=w402, "error in"=w406, "String Value"=w401, "name in"=w403, "Step in"=w405) -> ("error out"=w399:errorcluster, "Step out"=w400:variant)  [unwired: 3 in, 2 out]
      }
      n132 = Build Array(w394) -> (w398:variant[])
    }
    frame "JUMP" {
      (unwired) "StepPointer" ("source")
      (unwired) string[] ["Step Pointer"] ("source")
      # "JUMP\njump to step by name\n\narguments:\n(1) Step name (step pointer)"
      n133 = call-poly "variantCtrl.polymorphic.vi"("menu in (get)"=w410, "StepFunction"=type.StepFunction."_JUMP" ("Operation out"), "variant in"=w411) -> ("error out"=w412:errorcluster, "variant out"=w413:variant)  [unwired: 5 in, 2 out]
      n134 = call-poly "variantCtrl.polymorphic.vi"("menu in (get)"=w410, "error in"=w412, "String in"=w407, "stepElement in in"=w413) -> ("error out"=w408:errorcluster, "stepElement out"=w409:variant)  [unwired: 4 in, 2 out]
      n135 = Build Array(w409) -> (w415:variant[])
    }
    frame "COMPLETE" {
      # "COMPLETE\nSET PROC.RUNNING OFF\n\narguments:"
      n136 = call-poly "variantCtrl.polymorphic.vi"("menu in (get)"=w418, "StepFunction"=type.StepFunction."_COMPLETE" ("Operation out"), "variant in"=w419) -> ("error out"=w416:errorcluster, "variant out"=w417:variant)  [unwired: 5 in, 2 out]
      n137 = Build Array(w417) -> (w421:variant[])
    }
    frame "LOG-MESSAGE" {
      (unwired) "Message,File" ("source")
      (unwired) string[] ["Message", "File Pointer"] ("source")
      # "LOG-MESSAGE\nsave message log\n \narguments:\n(1) Output name\n(2) Output State (String formated). For digital outputs use \"A:B\" format where A is 0 or 1 representing the boolean state of digital output and B is timeout value in seconds, de-activating the output automatically\n(3) Path to *.rec file"
      n138 = call-poly "variantCtrl.polymorphic.vi"("menu in (get)"=w423, "StepFunction"=type.StepFunction."_LOG_MESSAGE" ("Operation out"), "variant in"=w432) -> ("error out"=w429:errorcluster, "variant out"=w430:variant)  [unwired: 5 in, 2 out]
      n139 = call-poly "variantCtrl.polymorphic.vi"("menu in (get)"=w423, "error in"=w429, "String in"=w428, "stepElement in in"=w430) -> ("error out"=w425:errorcluster, "stepElement out"=w427:variant)  [unwired: 4 in, 2 out]
      n140 = disable-structure shown="Enabled" {
        disable-tunnel: w427 -> [w439 w441]
        disable-tunnel: [w438 w441] -> w426
        disable-tunnel: w425 -> [w437 w440]
        disable-tunnel: [w436 w440] -> w424
        disable-tunnel: w423 -> [w435 _]
        disable-tunnel: w422 -> [w434 _]
        frame Disabled {
          n141 = call-poly "variantCtrl.polymorphic.vi"("menu(get)"=w435, "error in (no error)"=w437, "File Pointer in"=w434, "stepElement in"=w439) -> ("error out"=w436:errorcluster, "step\\element out"=w438:variant)  [unwired: 5 in, 1 out]
        }
        frame Enabled {
        }
      }
      n142 = Build Array(w426) -> (w433:variant[])
    }
    frame "LOG-REPORT" {
      (unwired) "File" ("source")
      (unwired) string[] ["File Pointer"] ("source")
      # "LOG-REPORT\nsave report log generated by previouse step.\n\narguments:\n(1) Output name\n(2) Output State (String formated). For digital outputs use \"A:B\" format where A is 0 or 1 representing the boolean state of digital output and B is timeout value in seconds, de-activating the output automatically\n(3) Path to *.rec file"
      n143 = call-poly "variantCtrl.polymorphic.vi"("menu in (get)"=w448, "StepFunction"=type.StepFunction."_LOG_LAST_REPORT" ("Operation out"), "variant in"=w449) -> ("error out"=w443:errorcluster, "variant out"=w444:variant)  [unwired: 5 in, 2 out]
      n144 = call-poly "variantCtrl.polymorphic.vi"("menu(get)"=w448, "error in (no error)"=w443, "File Pointer in"=w442, "stepElement in"=w444) -> ("error out"=w446:errorcluster, "step\\element out"=w447:variant)  [unwired: 5 in, 1 out]
      n145 = Build Array(w447) -> (w450:variant[])
    }
    frame "PROC-IS-COMPLETED" {
      (unwired) "ProcPointer" ("source")
      (unwired) string[] ["Proc Pointer"] ("source")
      # "PROC-COMPLETION-CHECK \ncheck if procedure is completed and go NEXT or jump otherwise\n\n arguments:\n(1) Procedure Pointer\n\ndescriptions: load"
      n146 = stacked-sequence {
        tunnel: [w466 _] -> w458
        tunnel: [_ w474] -> w457
        tunnel: w451 -> [w463 w473]
        tunnel: [w462 _] -> w456
        tunnel: [_ w472] -> w455
        tunnel: w453 -> [w461 _]
        tunnel: w452 -> [w460 w471]
        frame #0 {
          n147 = call-poly "variantCtrl.polymorphic.vi"("menu in (get)"=w460, "StepFunction"=type.StepFunction."PROC_COMPLETION_LOAD" ("Operation out"), "variant in"=w461) -> ("error out"=w469:errorcluster, "variant out"=w468:variant)  [unwired: 5 in, 2 out]
          n148 = call "proc.util.enumToStrStepVar.vi"("Step var"=typeStepVarients."stepProcPointer") -> ("String"=w465:string)  [unwired: 10 in]
          n149 = call-poly "variantCtrl.polymorphic.vi"("menu in (get)"=w460, "error in"=w469, "String Value"=w463, "name in"=w465, "Step in"=w468) -> ("error out"=w462:errorcluster, "Step out"=w466:variant)  [unwired: 3 in, 2 out]
        }
        frame #1 {
          n150 = call-poly "variantCtrl.polymorphic.vi"("menu in (get)"=w471, "StepFunction"=type.StepFunction."PROC_COMPLETION_CHECK" ("Operation out"), "variant in"=variant) -> ("error out"=w479:errorcluster, "variant out"=w478:variant)  [unwired: 5 in, 2 out]
          n151 = call "proc.util.enumToStrStepVar.vi"("Step var"=typeStepVarients."stepProcPointer") -> ("String"=w476:string)  [unwired: 10 in]
          n152 = call-poly "variantCtrl.polymorphic.vi"("menu in (get)"=w471, "error in"=w479, "String Value"=w473, "name in"=w476, "Step in"=w478) -> ("error out"=w472:errorcluster, "Step out"=w474:variant)  [unwired: 3 in, 2 out]
        }
      }
      n153 = Merge Errors(w456, w455) -> (w454:errorcluster)
      n154 = Build Array(w458, w457) -> (w459:variant[])
    }
    frame "PROC-LOAD" {
      (unwired) "ProcPointer" ("source")
      (unwired) string[] ["Proc Pointer"] ("source")
      n155 = call-poly "variantCtrl.polymorphic.vi"("menu in (get)"=w482, "StepFunction"=type.StepFunction."PROC_LOAD" ("Operation out"), "variant in"=w480) -> ("error out"=w488:errorcluster, "variant out"=w487:variant)  [unwired: 5 in, 2 out]
      n156 = call "proc.util.enumToStrStepVar.vi"("Step var"=typeStepVarients."stepProcPointer") -> ("String"=w484:string)  [unwired: 10 in]
      n157 = call-poly "variantCtrl.polymorphic.vi"("menu in (get)"=w482, "error in"=w488, "String Value"=w481, "name in"=w484, "Step in"=w487) -> ("error out"=w483:errorcluster, "Step out"=w489:variant)  [unwired: 3 in, 2 out]
      n158 = Build Array(w489) -> (w490:variant[])
    }
    frame "PROC-START" {
      (unwired) "ProcPointer" ("source")
      (unwired) string[] ["Proc Pointer"] ("source")
      n159 = call-poly "variantCtrl.polymorphic.vi"("menu in (get)"=w494, "StepFunction"=type.StepFunction."PROC_START" ("Operation out"), "variant in"=w491) -> ("error out"=w500:errorcluster, "variant out"=w499:variant)  [unwired: 5 in, 2 out]
      n160 = call "proc.util.enumToStrStepVar.vi"("Step var"=typeStepVarients."stepProcPointer") -> ("String"=w496:string)  [unwired: 10 in]
      n161 = call-poly "variantCtrl.polymorphic.vi"("menu in (get)"=w494, "error in"=w500, "String Value"=w492, "name in"=w496, "Step in"=w499) -> ("error out"=w495:errorcluster, "Step out"=w493:variant)  [unwired: 3 in, 2 out]
      n162 = Build Array(w493) -> (w501:variant[])
    }
    frame "PROC-STOP" {
      (unwired) "ProcPointer" ("source")
      (unwired) string[] ["Proc Pointer"] ("source")
      n163 = call-poly "variantCtrl.polymorphic.vi"("menu in (get)"=w504, "StepFunction"=type.StepFunction."PROC_STOP" ("Operation out"), "variant in"=w502) -> ("error out"=w510:errorcluster, "variant out"=w509:variant)  [unwired: 5 in, 2 out]
      n164 = call "proc.util.enumToStrStepVar.vi"("Step var"=typeStepVarients."stepProcPointer") -> ("String"=w506:string)  [unwired: 10 in]
      n165 = call-poly "variantCtrl.polymorphic.vi"("menu in (get)"=w504, "error in"=w510, "String Value"=w503, "name in"=w506, "Step in"=w509) -> ("error out"=w505:errorcluster, "Step out"=w511:variant)  [unwired: 3 in, 2 out]
      n166 = Build Array(w511) -> (w512:variant[])
    }
    frame "RECORD-MOVE" {
      # "\"RECORD-FILE-MOVE\" \nRename record file\n\narguments:\n(1) Input1 (uv sensor)\n(3) File1 (record uv)"
      n167 = disable-structure shown="Enabled" {
        disable-tunnel: w521 -> [w538 w540 _]
        disable-tunnel: w518 -> [w537 w539 _]
        disable-tunnel: w517 -> [w534 _ _]
        disable-tunnel: w516 -> [w533 _ _]
        disable-tunnel: w515 -> [w532 _ _]
        disable-tunnel: [w530 w541 _] -> w514
        frame Disabled {
          n168 = Build Array(w534, w533, w532) -> (w531:string[])
          n169 = Build Array(w538, w537) -> (w536:string[])
          n170 = call "util.DelimitedStringFromArray.vi"("params array in"=w531) -> ("delimited string out"=w529:string)  [unwired: 10 in]
          n171 = call "util.DelimitedStringFromArray.vi"("params array in"=w536) -> ("delimited string out"=w535:string)  [unwired: 10 in]
          n172 = Build Array(w535, w529) -> (w530:string[])
        }
        frame Enabled {
          n173 = Build Array(w540, w539) -> (w542:string[])
          n174 = call "util.DelimitedStringFromArray.vi"("params array in"=w542) -> ("delimited string out"=w541:string)  [unwired: 10 in]
        }
        frame Disabled {
        }
      }
      n175 = call-poly "variantCtrl.polymorphic.vi"("menu in (get)"=w522, "StepFunction"=type.StepFunction."_REC_MOVE" ("Operation out"), "variant in"=w520) -> ("error out"=w527:errorcluster, "variant out"=w526:variant)  [unwired: 5 in, 2 out]
      n176 = call "proc.util.enumToStrStepVar.vi"("Step var"=typeStepVarients."stepFilePointer") -> ("String"=w513:string)  [unwired: 10 in]
      n177 = call-poly "variantCtrl.polymorphic.vi"("menu in (get)"=w522, "error in"=w527, "String Value"=w514, "name in"=w513, "Step in"=w526) -> ("error out"=w523:errorcluster, "Step out"=w519:variant)  [unwired: 3 in, 2 out]
      n178 = Build Array(w519) -> (w528:variant[])
    }
    frame "IRR-CHECK" {
      # "\"IRR-CHECK\" \nCHECK IRRIGATION TIMING PARAMS AND ADD IRRIGATION DOSING INSTRUCTION"
      n179 = Decimal String To Number(string=w545) -> (number=w543:i32)  [unwired: 2 in, 1 out]
      n180 = call-poly "variantCtrl.polymorphic.vi"("menu in (get)"=w552, "StepFunction"=type.StepFunction."_IRR_CHECK" ("Operation out"), "variant in"=w553) -> ("error out"=w550:errorcluster, "variant out"=w549:variant)  [unwired: 5 in, 2 out]
      n181 = call "proc.util.enumToStrStepVar.vi"("Step var"=typeStepVarients."stepSeconds") -> ("String"=w544:string)  [unwired: 10 in]
      n182 = call-poly "variantCtrl.polymorphic.vi"("menu in (get)"=w552, "error in"=w550, "number"=w543, "name in"=w544, "variant in"=w549) -> ("error out"=w551:errorcluster, "variant out"=w546:variant)  [unwired: 3 in, 2 out]
      n183 = Merge Errors(w551) -> (w554:errorcluster)
      n184 = Build Array(w546) -> (w555:variant[])
    }
    frame "UNIT-CHECK" {
      n185 = disable-structure shown="Disabled" {
        disable-tunnel: w557 -> [w579 _]
        disable-tunnel: [w573 _] -> _
        disable-tunnel: [w572 _] -> _
        disable-tunnel: [w570 _] -> w556
        frame Disabled {
          n186 = Concatenate Strings("UNIT" ("string"), w579) -> (w577:string)
          n187 = Concatenate Strings("1:0" ("element")) -> (w574:string)
          n188 = Build Array(w577, w574) -> (w576:string[])
          n189 = call "build.flowToVarient.io-write.vi"("flow params"=w576) -> ("error out"=w571:errorcluster, "variant out"=w572:variant)  [unwired: 9 in]
          n190 = call "build.flow-to-inst.delay.vi"("error in"=w571) -> ("error out"=w570:errorcluster, "Array"=w573:variant[])  [unwired: 9 in]
        }
        frame Enabled {
        }
      }
      n191 = Fract/Exp String To Number(string=w557) -> (number=w559:dbl)  [unwired: 3 in, 1 out]
      n192 = call-poly "variantCtrl.polymorphic.vi"("menu in (get)"=w566, "StepFunction"=type.StepFunction."UNIT_CHECK" ("Operation out"), "variant in"=w567) -> ("error out"=w564:errorcluster, "variant out"=w563:variant)  [unwired: 5 in, 2 out]
      n193 = call "proc.util.enumToStrStepVar.vi"("Step var"=typeStepVarients."stepUnitIndex") -> ("String"=w558:string)  [unwired: 10 in]
      n194 = call-poly "variantCtrl.polymorphic.vi"("menu in (get)"=w566, "error in"=w564, "number"=w559, "name in"=w558, "variant in"=w563) -> ("error out"=w565:errorcluster, "variant out"=w560:variant)  [unwired: 3 in, 2 out]
      n195 = Merge Errors(w565, w556) -> (w568:errorcluster)
      n196 = Build Array(w560) -> (w569:variant[])
    }
    frame "OCS-CHECK" {
      n197 = call-poly "variantCtrl.polymorphic.vi"("menu in (get)"=w583, "StepFunction"=type.StepFunction."_OCS_CHECK" ("Operation out"), "variant in"=w584) -> ("error out"=w582:errorcluster, "variant out"=w581:variant)  [unwired: 5 in, 2 out]
      n198 = Build Array(w581) -> (w585:variant[])
    }
    frame "OCS-RECORD" {
      n199 = call-poly "variantCtrl.polymorphic.vi"("menu in (get)"=w589, "StepFunction"=type.StepFunction."_OCS_RECORD" ("Operation out"), "variant in"=w590) -> ("error out"=w588:errorcluster, "variant out"=w587:variant)  [unwired: 5 in, 2 out]
      n200 = Build Array(w587) -> (w591:variant[])
    }
    frame "SCHEDULER" {
      # "\"SCHEDULER\"  (ENCODED CLUSTER TO STRING)\nNOTE: THIS STEP REQUIRES A UNIQE CLUSTER OF TYPE AND PAIR ARRAY AND THIS STEP IS CONFIGURED PROGRAMATICALLY IN ICC DEVICE CONFIGURATOR AND NEVER MANUALLY IN BUILDER"
      n201 = call-poly "variantCtrl.polymorphic.vi"("menu in (get)"=w600, "StepFunction"=type.StepFunction."_SCHEDULE" ("Operation out"), "variant in"=w601) -> ("error out"=w598:errorcluster, "variant out"=w597:variant)  [unwired: 5 in, 2 out]
      n202 = call "proc.util.enumToStrStepVar.vi"("Step var"=typeStepVarients."stepStrReg") -> ("String"=w593:string)  [unwired: 10 in]
      n203 = call-poly "variantCtrl.polymorphic.vi"("menu in (get)"=w600, "error in"=w598, "String Value"=w592, "name in"=w593, "Step in"=w597) -> ("error out"=w599:errorcluster, "Step out"=w594:variant)  [unwired: 3 in, 2 out]
      n204 = Merge Errors(w599) -> (w602:errorcluster)
      n205 = Build Array(w594) -> (w603:variant[])
    }
    frame "UNIT-SAMPLE" {
      n206 = disable-structure shown="Disabled" {
        disable-tunnel: w605 -> [w627 _]
        disable-tunnel: [w621 _] -> _
        disable-tunnel: [w620 _] -> _
        disable-tunnel: [w618 _] -> w604
        frame Disabled {
          n207 = Concatenate Strings("UNIT" ("string"), w627) -> (w625:string)
          n208 = Concatenate Strings("1:0" ("element")) -> (w622:string)
          n209 = Build Array(w625, w622) -> (w624:string[])
          n210 = call "build.flowToVarient.io-write.vi"("flow params"=w624) -> ("error out"=w619:errorcluster, "variant out"=w620:variant)  [unwired: 9 in]
          n211 = call "build.flow-to-inst.delay.vi"("error in"=w619) -> ("error out"=w618:errorcluster, "Array"=w621:variant[])  [unwired: 9 in]
        }
        frame Enabled {
        }
      }
      n212 = Fract/Exp String To Number(string=w605) -> (number=w607:dbl)  [unwired: 3 in, 1 out]
      n213 = call-poly "variantCtrl.polymorphic.vi"("menu in (get)"=w614, "StepFunction"=type.StepFunction."UNIT_SAMPLE" ("Operation out"), "variant in"=w615) -> ("error out"=w612:errorcluster, "variant out"=w611:variant)  [unwired: 5 in, 2 out]
      n214 = call "proc.util.enumToStrStepVar.vi"("Step var"=typeStepVarients."stepUnitIndex") -> ("String"=w606:string)  [unwired: 10 in]
      n215 = call-poly "variantCtrl.polymorphic.vi"("menu in (get)"=w614, "error in"=w612, "number"=w607, "name in"=w606, "variant in"=w611) -> ("error out"=w613:errorcluster, "variant out"=w608:variant)  [unwired: 3 in, 2 out]
      n216 = Merge Errors(w613, w604) -> (w616:errorcluster)
      n217 = Build Array(w608) -> (w617:variant[])
    }
    frame "UNIT-DOSE" {
      (unwired) "seconds" ("source")
      # "\"UNIT-DOSE\" (unitIndex, output, dosingTime)"
      n218 = Decimal String To Number(string=w629) -> (number=w639:i32)  [unwired: 2 in, 1 out]
      n219 = Decimal String To Number(string=w645) -> (number=w630:i32)  [unwired: 2 in, 1 out]
      n220 = call-poly "variantCtrl.polymorphic.vi"("menu in (get)"=w628, "StepFunction"=type.StepFunction."UNIT_DOSE" ("Operation out"), "variant in"=w648) -> ("error out"=w644:errorcluster, "variant out"=w643:variant)  [unwired: 5 in, 2 out]
      n221 = call "proc.util.enumToStrStepVar.vi"("Step var"=typeStepVarients."stepUnitIndex") -> ("String"=w640:string)  [unwired: 10 in]
      n222 = call "proc.util.enumToStrStepVar.vi"("Step var"=typeStepVarients."stepIoPointer") -> ("String"=w637:string)  [unwired: 10 in]
      n223 = call "proc.util.enumToStrStepVar.vi"("Step var"=typeStepVarients."stepSeconds") -> ("String"=w631:string)  [unwired: 10 in]
      n224 = call-poly "variantCtrl.polymorphic.vi"("menu in (get)"=w628, "error in"=w644, "number"=w639, "name in"=w640, "variant in"=w643) -> ("error out"=w635:errorcluster, "variant out"=w636:variant)  [unwired: 3 in, 2 out]
      n225 = call-poly "variantCtrl.polymorphic.vi"("menu in (get)"=w628, "error in"=w635, "String Value"=w646, "name in"=w637, "Step in"=w636) -> ("error out"=w633:errorcluster, "Step out"=w634:variant)  [unwired: 3 in, 2 out]
      n226 = call-poly "variantCtrl.polymorphic.vi"("menu in (get)"=w628, "error in"=w633, "number"=w630, "name in"=w631, "variant in"=w634) -> ("error out"=w649:errorcluster, "variant out"=w650:variant)  [unwired: 3 in, 2 out]
      n227 = Build Array(w650) -> (w647:variant[])
    }
    frame Default {
      (unwired) "" ("source")
      w654 = errorcluster {"status"=TRUE, "code"=-1, "source"=""}  # error
      n228 = Format Into String(format string="%s is unsupported", w655) -> (resulting string=w653:string)  [unwired: 2 in, 1 out]
      n229 = Bundle By Name(cluster=w654, "source"=w653) -> (w652:errorcluster)
    }
  }
  "error out" <- w25
  "instructions out" <- w26
  n230 = case shown="True" w5 {
    tunnel: w4 -> [_ w657]
    tunnel: [_ w657] -> w3
    frame False {
    }
    frame True {
    }
  }
  "format string" <- w3
